vi "ABRE ARCHIVO.vi"(0 "File Path Control":path, 11 "error in (no error)":errorcluster) -> (3 "Número de datos":i32, 4 "EJE X":dbl[](array[numeric]), 6 "EJE Y":dbl[](array[numeric]), 8 "Ángulo máximo":dbl, 10 "Ángulo mínimo":dbl, 15 "error out":errorcluster)   [LabVIEW 2025, in "Control de MaP.lvlib"]
uses:
  Control de MaP.lvlib
  <vilib>/Utility/file.llb/Read From Spreadsheet File (DBL).vi
panel:
  out "EJE X y Y":dbl[][](array[numeric])
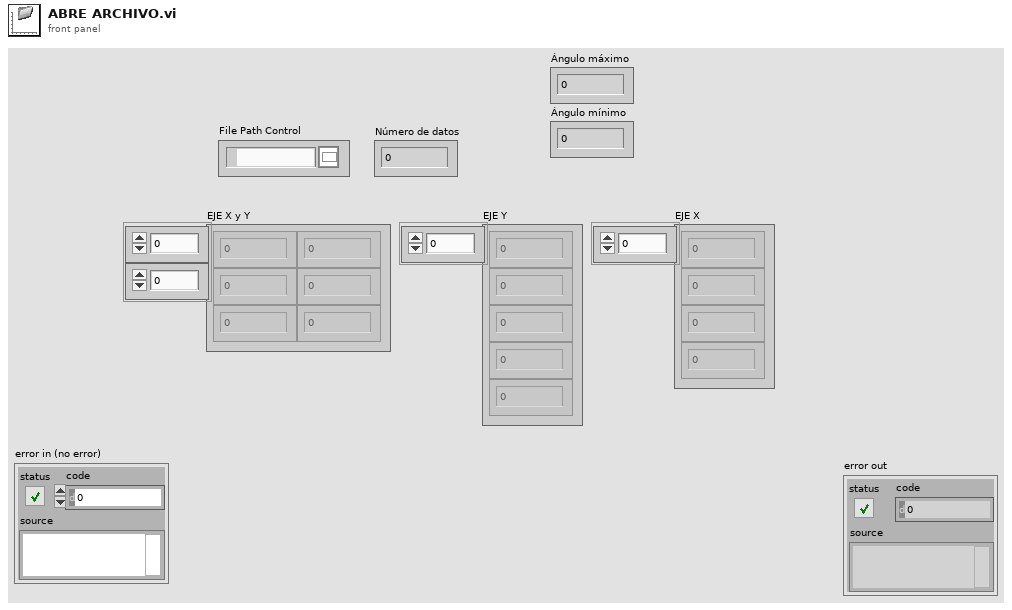
[diagram p1: front panel]
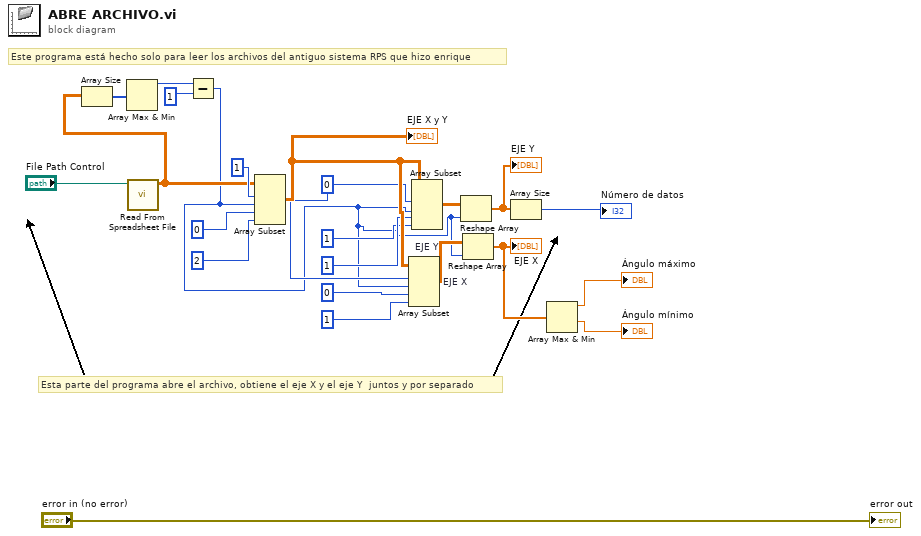
[diagram p0: block diagram]
diagram:
  w17 = 0 ("index")
  # "Esta parte del programa abre el archivo, obtiene el eje X y el eje Y  juntos y por separado"
  # "Este programa está hecho solo para leer los archivos del antiguo sistema RPS que hizo enrique"
  n1 = call-poly <vilib>:"Read From Spreadsheet File.vi"("file path (dialog if empty)"="File Path Control") -> ("all rows"=w5:dbl[][])  [unwired: 6 in, 4 out]
  n2 = Array Size(array=w5) -> (size(s)=w4:i32[])
  n3 = Array Max & Min(array=w4) -> (max value=w3:i32)  [unwired: 3 out]
  n4 = Subtract(x=w3, y=1) -> (x-y=w1:i32)
  n5 = Array Subset(array=w5, index (row)=1 ("index"), length (row)=w1, index (col)=0 ("index"), length (col)=2 ("length")) -> (w20:dbl[][])
  "EJE X y Y" <- w20
  n6 = Array Subset "EJE X"(array=w20, index (row)=w17, length (row)=w1, index (col)=0 ("index"), length (col)=1 ("length")) -> (w14:dbl[][])
  n7 = Array Subset "EJE Y"(array=w20, index (row)=w17, length (row)=w1, index (col)=1 ("index"), length (col)=1 ("length")) -> (w13:dbl[][])
  n8 = Reshape Array(w13, w1) -> (w11:dbl[])
  "EJE Y" <- w11
  n9 = Reshape Array(w14, w1) -> (w7:dbl[])
  "EJE X" <- w7
  n10 = Array Size(array=w11) -> (size(s)=→"Número de datos":i32)
  n11 = Array Max & Min(array=w7) -> (max value=→"Ángulo máximo":dbl, min value=→"Ángulo mínimo":dbl)  [unwired: 2 out]
  "error out" <- "error in (no error)"
